vi "VI Tree - lvdata.vi"() -> ()   [LabVIEW 2020]
uses:
  Type Descriptor Enumeration.ctl
  Type Descriptor Header.ctl
  Refnum Code.ctl
  Base Units.ctl
  Physical Units.ctl
  Type Descriptor.ctl
  Waveform Subtype Enum.ctl
  Refnum Subtype Enum.ctl
  LVData/Type Descriptor/TD.lvclass
  LVData/Type Descriptor/ArrayTD/Array.lvclass
  LVData/Type Descriptor/Cluster/Cluster.lvclass
  0ad02e67-9589-400a-9d5c-190c99c4dee1.vi
  Get Collection Subtype.vi
  openg_variant.lvlib
  LVData/variant.lvclass
  LVData/DataString/DataString.lvclass
  variant.lvlib
  C:/projects/OpenG-Variant-Data-Library/source/library/LVData/Type Descriptor/TD.lvclass
  C:/projects/OpenG-Variant-Data-Library/source/library/Bytes/Bytes.lvclass
  C:/projects/OpenG-Variant-Data-Library/source/library/LVData/Type Descriptor/Cluster/Cluster.lvclass
panel:
  out "Array Type Descriptor":refnum<class "Array.lvclass">
  out "TypeDescriptor":refnum<class "TD.lvclass">
  in  "Refnum Subtype Enum":T1 format="%.0x"
  in  "Waveform Subtype Enum":T2 format="%.0x"
  in  "Type Descriptor":T3
  in  "Physical Units":T4
  in  "Base Units":T5
  in  "Refnum Code":T6
  out "Type Descriptor Header":T7 {"type" format="%.0x"}
  in  "Type Descriptor Enumeration":T8 format="%.0x"
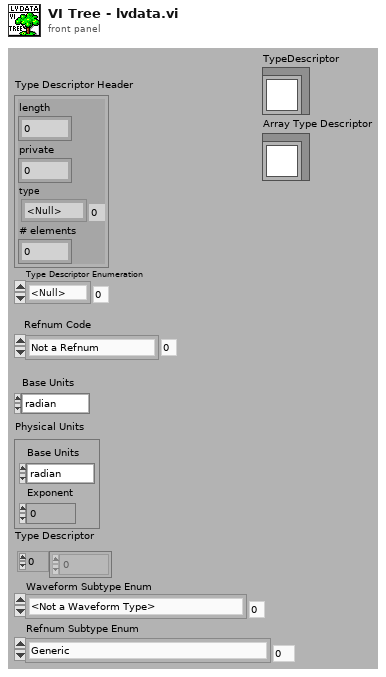
[diagram p1: front panel]
types:
  T1 = typedef "openg_variant.lvlib/Refnum Subtype Enum.ctl" = enum8{"Generic", "Datalog File Refnum", "Byte Stream File Refnum", "Device Refnum", "Occurence Refnum", "TCP Connection Refnum", "VISA Refnum (Obsolete)", "Automation Renum", "VI Server Refnum", "Menu Refnum", "IVI Refnum (Obsolete)", "IMAQ Session", "0x0C", "Datasocket Refnum", "VISA Resource", "IVI Logical Name", "UDP Connection Refnum", "Notifier Refnum", "Queue Refnum", "IrDA Refnum", "Hardware Plugin Refnum", "Hardware Plugin Tag Refnum", "DAQmx Refnum", "Event Registration Refnum", ".NET Refnum", "User Event Refnum", "0x1A", "Event Callback", "0x1C", "0x1D", "LabVIEW Class Instance", "Bluetooth", "Data Value References", "RT FIFO", "TDM Streaming"}
  T2 = typedef "openg_variant.lvlib/Waveform Subtype Enum.ctl" = enum8{"<Not a Waveform Type>", "0x01", "Analog 16-bit signed", "Analog Double-Precision", "0x04", "Analog Single Precision", "Timestamp", "Digital Data", "Digital Waveform", "Dynamic Data", "Analog Extended-Precision", "Analog 8-bit unsigned", "Analog 16-bit unsigned", "Analog 32-bit unsigned", "Analog 8-bit signed", "Analog 32-bit signed", "Analog Complex Single-Precision", "Analog Complex Double-Precision", "Analog Complex Extended Precision", "Analog 64-bit signed", "Analog 64-bit unsigned"}
  T3 = typedef "openg_variant.lvlib/Type Descriptor.ctl" = i16[]
  T4 = typedef "openg_variant.lvlib/Physical Units.ctl" = cluster{"Base Units":enum16{"radian", "steradian", "second", "meter", "kilogram", "ampere", "kelvin", "mole", "candela"}, "Exponent":i16}
  T5 = typedef "openg_variant.lvlib/Base Units.ctl" = enum16{"radian", "steradian", "second", "meter", "kilogram", "ampere", "kelvin", "mole", "candela"}
  T6 = typedef "openg_variant.lvlib/Refnum Code.ctl" = enum16{"Not a Refnum", "Datalog File", "Byte Stream File", "0x03", "Occurence", "TCP", "0x06", "ActiveX", "Generic VI Server Class", "Menu", "0x0A", "IMAQ Session", "0x0C", "0x0D", "VISA", "IVI", "UDP"}
  T7 = typedef "openg_variant.lvlib/Type Descriptor Header.ctl" = cluster{"length":u16, "private":u8, "type":T8, "# elements":u16}
  T8 = typedef "openg_variant.lvlib/Type Descriptor Enumeration.ctl" = enum8{"<Null>", "I8", "I16", "I32", "I64", "U8", "U16", "U32", "U64", "SGL", "DBL", "EXT", "CSG", "CDB", "CXT", "0x0F", "0x10", "0x11", "0x12", "0x13", "0x14", "Enum U8", "Enum U16", "Enum U32", "Enum U64", "SGL PQ", "DBL PQ", "EXT PQ", "CSG PQ", "CDB PQ", "CXT PQ", "0x1F", "0x20", "Boolean", "0x22", "0x23", "0x24", "0x25", "0x26", "0x27", "0x28", "0x29", "0x2A", "0x2B", "0x2C", "0x2D", "0x2E", "0x2F", "String", "0x31", "Path", "Pict", "0x34", "0x35", "0x36", "DAQ", "0x38", "0x39", "0x3A", "0x3B", "0x3C", "0x3D", "0x3E", "0x3F", "Array", "0x41", "0x42", "0x43", "0x44", "0x45", "0x46", "0x47", "0x48", "0x49", "0x4A", "0x4B", "0x4C", "0x4D", "0x4E", "0x4F", "Cluster", "0x51", "0x52", "Variant", "Waveform", "0x55", "0x56", "0x57", "0x58", "0x59", "0x5A", "0x5B", "0x5C", "0x5D", "0x5E", "Fixed Point", "0x60", "0x61", "0x62", "0x63", "0x64", "0x65", "0x66", "0x67", "0x68", "0x69", "0x6A", "0x6B", "0x6C", "0x6D", "0x6E", "0x6F", "Refnum", "0x71", "0x72", "Set Collection", "Map Collection"}
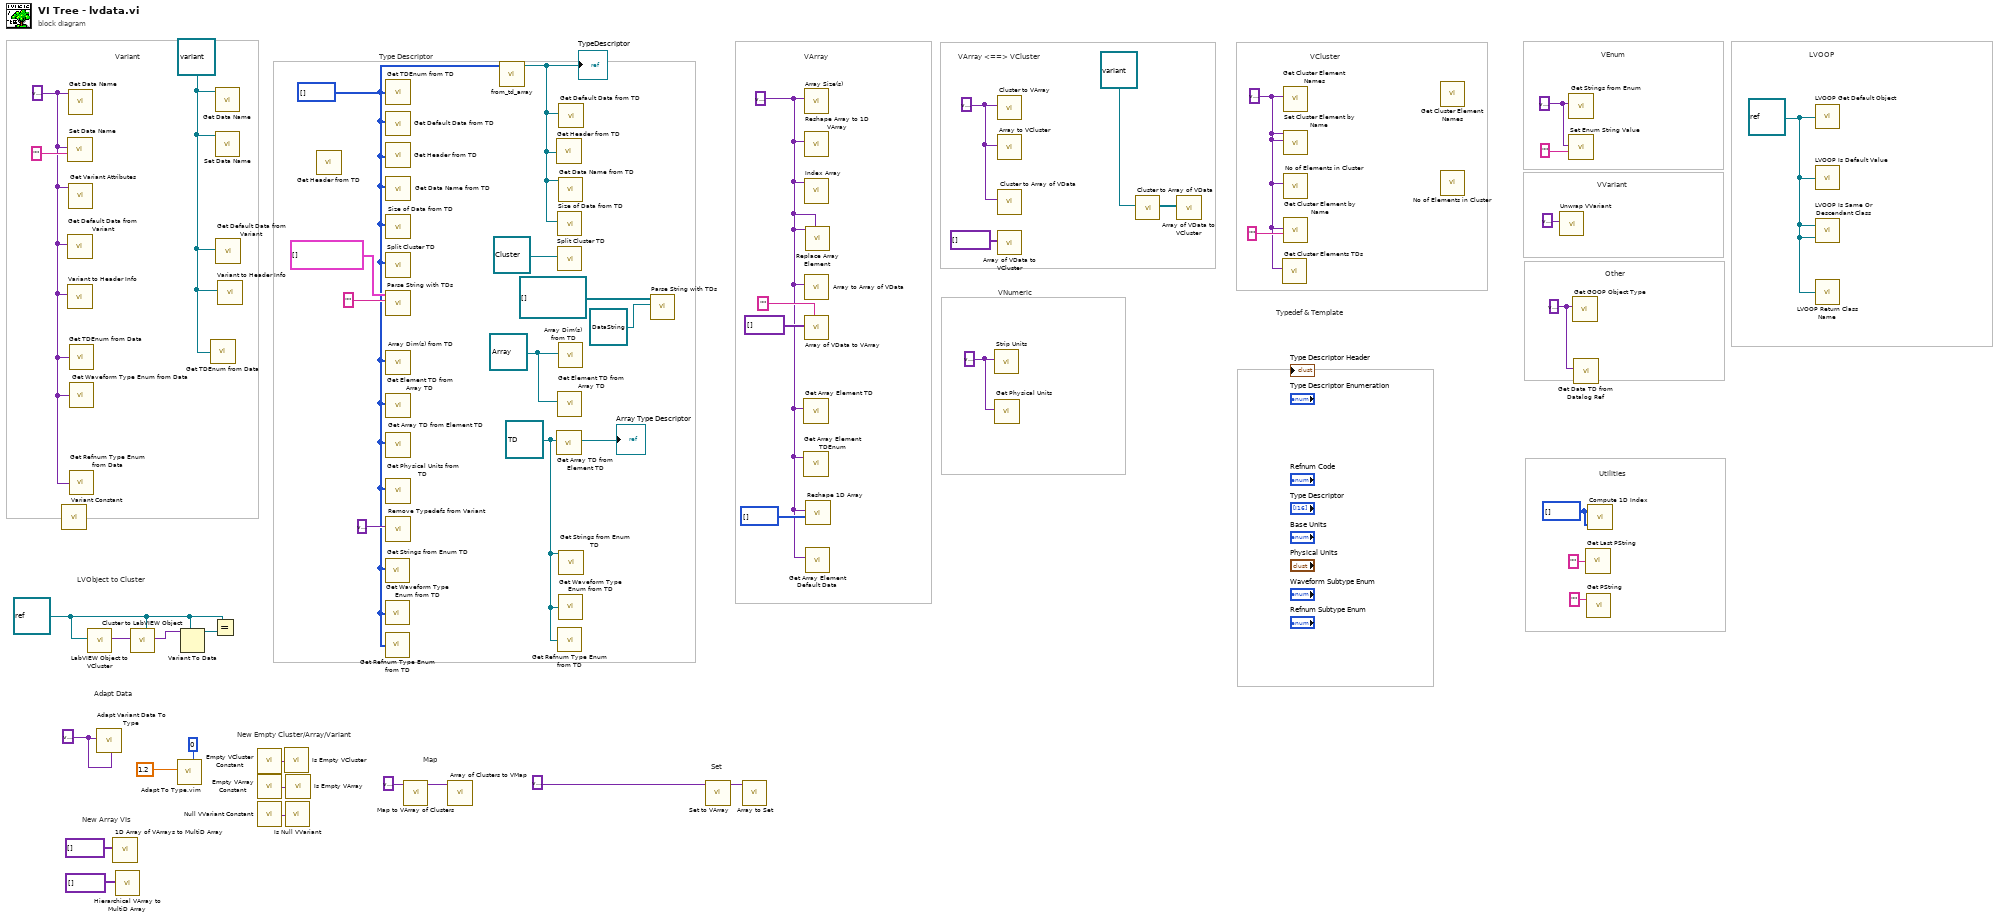
[diagram p0: block diagram]
diagram:
  w2 = refnum<class "variant.lvclass"> refnum ("variant.lvlib:variant.lvclass")
  w1 = refnum<class "TD.lvclass"> refnum ("Element Type Descriptor")
  w9 = refnum<class "Array.lvclass"> refnum ("lvdata.lvlib:ArrayTD.lvclass")
  w23 = variant ("Type and Defaults")
  w24 = refnum<class> refnum ("LabVIEW Object")
  w28 = refnum<class> refnum ("Object")
  w34 = variant ("Number or 1D array with units")
  w30 = variant ("Enum")
  w33 = variant ("Cluster")
  w32 = variant ("Cluster")
  w48 = u32[] [] ("Indices")
  w11 = T3 [] ("Type Descriptor")
  w31 = variant ("GOOP Refnum")
  w35 = variant ("Array")
  w29 = variant ("Data")
  # "New Empty Cluster/Array/Variant"
  # "New Array VIs"
  # "Adapt Data"
  # "Set"
  # "Map"
  # "LVObject to Cluster"
  # "LVOOP"
  # "VVariant"
  # "VNumeric"
  # "Other"
  # "Type Descriptor"
  # "Typedef & Template"
  # "Variant"
  # "Utilities"
  # "VEnum"
  # "VArray <==> VCluster"
  # "VCluster"
  # "VArray"
  n1 = call "Variant Constant.vi"() -> ()  [unwired: 1 in]
  n2 = call "Set Data Name.vi"("Data Name"="", "Data"=w29) -> ()  [unwired: 8 in, 2 out]
  n3 = call "Get Default Data from Variant.vi"("Variant"=w29) -> ()  [unwired: 9 in, 2 out]
  n4 = call "Variant to Header Info.vi"("Variant"=w29) -> ()  [unwired: 3 in, 3 out]
  n5 = call "Get Data Name.vi"("Data"=w29) -> ()  [unwired: 8 in, 3 out]
  n6 = call "Get Variant Attributes.vi"("Variant"=w29) -> ()  [unwired: 3 in, 4 out]
  n7 = call "Get TDEnum from Data.vi"("Data"=w29) -> ()  [unwired: 4 in, 1 out]
  n8 = call "Get Waveform Type Enum from Data.vi"("Data"=w29) -> ()  [unwired: 4 in, 1 out]
  n9 = call "Get Refnum Type Enum from Data.vi"("Data"=w29) -> ()  [unwired: 4 in, 1 out]
  n10 = call "LabVIEW Object to VCluster.vi"("LabVIEW Object"=w24) -> ("VCluster"=w27:variant)  [unwired: 9 in, 1 out]
  n11 = call "Adapt Variant Data To Type.vi"("Type and Defaults"=w23, "Variant in"=w23) -> ()  [unwired: 8 in, 2 out]
  n12 = call "1D Array of VArrays to MultiD Array.vi"("Array of VArrays"=variant[] [] ("1D Array of VData")) -> ()  [unwired: 9 in, 2 out]
  n13 = call "Hierarchical VArray to MultiD Array.vi"("Hierarchical Array"=variant[] [] ("1D Array of VData")) -> ()  [unwired: 9 in, 2 out]
  n14 = call "Cluster to LabVIEW Object.vi"("VObject Type"=w24, "VCluster"=w27) -> ("VObject out"=w26:variant)  [unwired: 8 in, 1 out]
  n15 = call "Adapt To Type.vim"("type and defaults"=0, "data in"=1.2) -> ()  [unwired: 8 in, 2 out]
  n16 = Variant To Data(type=w24, Variant=w26) -> (data=w25:refnum<class>)  [unwired: 1 in, 1 out]
  n17 = call "Get TDEnum from Data.vi"("Data"=w2) -> ()  [unwired: 4 in, 1 out]
  n18 = Equal?(x=w24, y=w25) -> ()  [unwired: 1 out]
  n19 = call "Get Data Name.vi"("Data"=w2) -> ()  [unwired: 8 in, 3 out]
  n20 = call "Set Data Name.vi"("LVData in"=w2) -> ()  [unwired: 9 in, 2 out]
  n21 = call "Get Default Data from Variant.vi"("Variant"=w2) -> ()  [unwired: 9 in, 2 out]
  n22 = call "Variant to Header Info.vi"("Variant"=w2) -> ()  [unwired: 3 in, 3 out]
  n23 = call "Empty VCluster Constant.vi"() -> ("Empty Cluster"=w18:variant)
  n24 = call "Empty VArray Constant.vi"() -> ("Empty Cluster"=w19:variant)
  n25 = call "Null VVariant Constant.vi"() -> ("Null VVariant"=w20:variant)
  n26 = call "Is Empty VCluster.vi"("Variant"=w18) -> ()  [unwired: 1 out]
  n27 = call "Is Null VVariant.vi"("Variant"=w20) -> ()  [unwired: 1 out]
  n28 = call "Is Empty VArray.vi"("Variant"=w19) -> ()  [unwired: 1 out]
  n29 = call "Get Header from TD.vi"() -> ()  [unwired: 1 in, 1 out]
  n30 = call "Get Strings from Enum TD.vi"("Type Descriptor"=w11) -> ()  [unwired: 8 in, 3 out]
  n31 = call "Get Waveform Type Enum from TD.vi"("Type Descriptor"=w11) -> ()  [unwired: 4 in, 1 out]
  n32 = call "Get Refnum Type Enum from TD.vi"("Type Descriptor"=w11) -> ()  [unwired: 4 in, 1 out]
  n33 = call "Get TDEnum from TD.vi"("Type Descriptor"=w11) -> ()  [unwired: 4 in, 1 out]
  n34 = call "Get Default Data from TD.vi"("Type Descriptor"=w11) -> ()  [unwired: 9 in, 2 out]
  n35 = call "Get Header from TD.vi"("Type Descriptor"=w11) -> ()  [unwired: 1 out]
  n36 = call "Get Data Name from TD.vi"("Type Descriptor"=w11) -> ()  [unwired: 9 in, 2 out]
  n37 = call "Size of Data from TD.vi"("Type Descriptor"=w11) -> ()  [unwired: 9 in, 2 out]
  n38 = call "Split Cluster TD.vi"("Type Descriptor"=w11) -> ()  [unwired: 9 in, 2 out]
  n39 = call "Parse String with TDs.vi"("Data string"="", "Type Descriptors"=cluster{"Type Descriptor":T3}[] []) -> ()  [unwired: 7 in, 3 out]
  n40 = call "Array Dim(s) from TD.vi"("Array Type Descriptor"=w11) -> ()  [unwired: 9 in, 2 out]
  n41 = call "Get Element TD from Array TD.vi"("Array Type Descriptor"=w11) -> ()  [unwired: 9 in, 2 out]
  n42 = call "Get Array TD from Element TD.vi"("Element Type Descriptor"=w11) -> ()  [unwired: 9 in, 2 out]
  n43 = call "Get Physical Units from TD.vi"("Float or Array Type Descriptor"=w11) -> ()  [unwired: 9 in, 2 out]
  n44 = call "Remove Typedefs from Variant.vi"("Variant with typedefs"=variant) -> ()  [unwired: 9 in, 2 out]
  n45 = call "Map to VArray of Clusters.vi"("Map"=variant ("Data")) -> ("Array of Clusters (key-value)"=w15:variant)  [unwired: 9 in, 1 out]
  n46 = call "Array of Clusters to VMap.vi"("Array of Clusters (key-value)"=w15) -> ()  [unwired: 9 in, 2 out]
  n47 = call "from_td_array.vi"("type descriptor array"=w11) -> ("TypeDescriptor out"=w3:refnum<class "TD.lvclass">)  [unwired: 9 in, 1 out]
  "TypeDescriptor" <- w3
  n48 = call "Get Header from TD.vi"("TypeDescriptor"=w3) -> ()  [unwired: 1 out]
  n49 = call "Get Array TD from Element TD.vi"("Element Type Descriptor"=w1) -> ("Array Type Descriptor"=→"Array Type Descriptor":refnum<class "Array.lvclass">)  [unwired: 9 in, 1 out]
  n50 = call "Size of Data from TD.vi"("TypeDescriptor"=w3) -> ()  [unwired: 9 in, 2 out]
  n51 = call "Split Cluster TD.vi"("Cluster TD"=refnum<class "Cluster.lvclass"> refnum ("ClusterTD")) -> ()  [unwired: 9 in, 2 out]
  n52 = call "Get Element TD from Array TD.vi"("Array Type Descriptor"=w9) -> ()  [unwired: 9 in, 2 out]
  n53 = call "Get Refnum Type Enum from TD.vi"("Type Descriptor"=w1) -> ()  [unwired: 4 in, 1 out]
  n54 = call "Get Data Name from TD.vi"("TypeDescriptor"=w3) -> ()  [unwired: 8 in, 3 out]
  n55 = call "Array Dim(s) from TD.vi"("Array Type Descriptor"=w9) -> ()  [unwired: 9 in, 2 out]
  n56 = call "Get Waveform Type Enum from TD.vi"("Type Descriptor"=w1) -> ()  [unwired: 4 in, 1 out]
  n57 = call "Get Default Data from TD.vi"("Type Descriptor"=w3) -> ()  [unwired: 9 in, 2 out]
  n58 = call "Get Strings from Enum TD.vi"("Type Descriptor"=w1) -> ()  [unwired: 7 in, 4 out]
  n59 = call "Parse String with TDs.vi"("DataString"=refnum<class "DataString.lvclass"> refnum, "Type Descriptors"=refnum<class "TD.lvclass">[] []) -> ()  [unwired: 7 in, 3 out]
  n60 = call "Set to VArray.vi"("Set"=variant ("Data")) -> ("Array"=w14:variant)  [unwired: 9 in, 1 out]
  n61 = call "Array to Set.vi"("Array"=w14) -> ()  [unwired: 9 in, 2 out]
  n62 = call "Get Array Element TD.vi"("Array"=w35) -> ()  [unwired: 9 in, 2 out]
  n63 = call "Get Array Element TDEnum.vi"("Array"=w35) -> ()  [unwired: 9 in, 2 out]
  n64 = call "Array Size(s).vi"("Array"=w35) -> ()  [unwired: 8 in, 3 out]
  n65 = call "Reshape Array to 1D VArray.vi"("MultiD Array"=w35) -> ()  [unwired: 8 in, 3 out]
  n66 = call "Index Array.vi"("MultiD Array"=w35) -> ()  [unwired: 9 in, 2 out]
  n67 = call "Array to Array of VData.vi"("MultiD Array"=w35) -> ()  [unwired: 9 in, 2 out]
  n68 = call "Array of VData to VArray.vi"("Array Name"="", "1D Array of VData"=variant[] []) -> ()  [unwired: 8 in, 2 out]
  n69 = call "Replace Array Element.vi"("New Element"=w35, "MultiD Array"=w35) -> ()  [unwired: 8 in, 2 out]
  n70 = call "Get Array Element Default Data.vi"("Array"=w35) -> ()  [unwired: 9 in, 2 out]
  n71 = call "Reshape 1D Array.vi"("Size(s)"=u32[] [], "1D Array"=w35) -> ()  [unwired: 8 in, 2 out]
  n72 = call "Strip Units.vi"("Number or 1D array with units"=w34) -> ()  [unwired: 9 in, 2 out]
  n73 = call "Get Physical Units.vi"("Float or Array of Floats"=w34) -> ()  [unwired: 9 in, 2 out]
  n74 = call "Cluster to VArray.vi"("Cluster"=w33) -> ()  [unwired: 9 in, 2 out]
  n75 = call "Array to VCluster.vi"("Array"=w33) -> ()  [unwired: 9 in, 2 out]
  n76 = call "Cluster to Array of VData.vi"("Cluster"=w33) -> ()  [unwired: 9 in, 2 out]
  n77 = call "Array of VData to VCluster.vi"("Array"=variant[] []) -> ()  [unwired: 9 in, 2 out]
  n78 = call "Cluster to Array of VData.vi"("Cluster"=refnum<class "variant.lvclass"> refnum ("variant.lvlib:variant.lvclass")) -> ("Array of VData"=w6:refnum<class "variant.lvclass">[])  [unwired: 9 in, 1 out]
  n79 = call "Array of VData to VCluster.vi"("Array"=w6) -> ()  [unwired: 9 in, 2 out]
  n80 = call "Get Cluster Elements TDs.vi"("Cluster"=w32) -> ()  [unwired: 9 in, 2 out]
  n81 = call "Get Cluster Element Names.vi"("Cluster"=w32) -> ()  [unwired: 9 in, 2 out]
  n82 = call "Set Cluster Element by Name.vi"("New Element Value"=w32, "Cluster"=w32) -> ()  [unwired: 7 in, 3 out]
  n83 = call "No of Elements in Cluster.vi"("Cluster"=w32) -> ()  [unwired: 9 in, 2 out]
  n84 = call "Get Cluster Element by Name.vi"("Element Name"="", "Cluster"=w32) -> ()  [unwired: 7 in, 3 out]
  n85 = call "Get Cluster Element Names.vi"() -> ()  [unwired: 9 in, 3 out]
  n86 = call "No of Elements in Cluster.vi"() -> ()  [unwired: 10 in, 2 out]
  n87 = call "Unwrap VVariant.vi"("VVariant"=variant) -> ()  [unwired: 9 in, 2 out]
  n88 = call "Get Strings from Enum.vi"("Enum"=w30) -> ()  [unwired: 7 in, 4 out]
  n89 = call "Set Enum String Value.vi"("String Value"="", "Default Enum Value"=w30) -> ()  [unwired: 8 in, 2 out]
  n90 = call "Get GOOP Object Type.vi"("GOOP Refnum"=w31) -> ()  [unwired: 9 in, 2 out]
  n91 = call "Get Data TD from Datalog Ref.vi"("Datalog Refnum"=w31) -> ()  [unwired: 9 in, 2 out]
  n92 = call "Get Last PString.vi"("String"="") -> ()  [unwired: 2 out]
  n93 = call "Get PString.vi"("String"="") -> ()  [unwired: 1 in, 2 out]
  n94 = call "Compute 1D Index.vi"("Size(s)"=w48, "Indices"=w48) -> ()  [unwired: 1 out]
  n95 = call "LVOOP Get Default Object.vi"("Object"=w28) -> ()  [unwired: 1 out]
  n96 = call "LVOOP Is Default Value.vi"("Object"=w28) -> ()  [unwired: 1 out]
  n97 = call "LVOOP Is Same Or Descendant Class.vi"("Possible Descendant Object"=w28, "Object"=w28) -> ()  [unwired: 1 out]
  n98 = call "LVOOP Return Class Name.vi"("Object"=w28) -> ()  [unwired: 3 out]
